vi "Handle Web service.vi"(7 "LabVIEW Web Service Request 2":refnum<class "Web Request.lvclass">, 11 "Server Name":string="3 phase testbench") -> ()   [LabVIEW 2025, in "MCP Server.lvlib"]
doc: "Use this VI in your LabVIEW Webservice inside a POST Method of any name. Just connect the Web Service reference, and the mcp server toolkit will handle all requests coming in through this method."
uses:
  MCP Server.lvlib
  <vilib>/wsapi/Web Request.lvclass
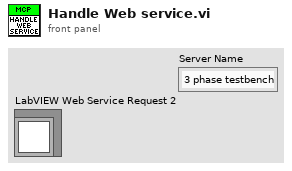
[diagram p1: front panel]
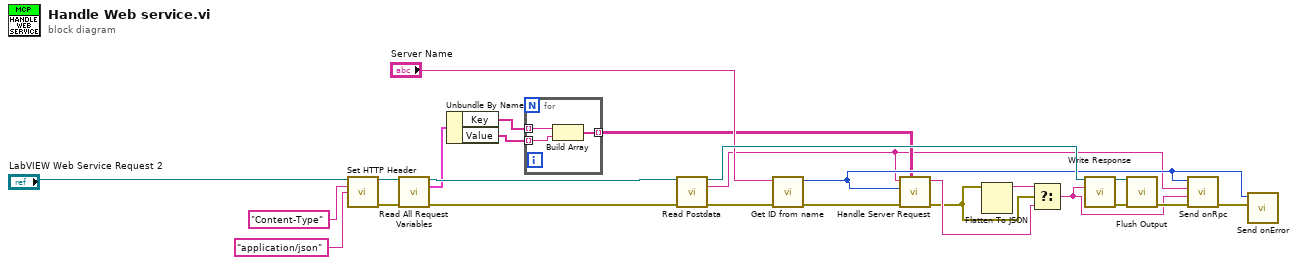
[diagram p0: block diagram]
diagram:
  n1 = call <vilib>:"Set HTTP Header.vi"("LabVIEW Web Service Request"="LabVIEW Web Service Request 2", "header"="Content-Type", "header value"="application/json") -> ("LabVIEW Web Service Request out"=w6:refnum<class "Web Request.lvclass">, "error out"=w9:errorcluster)  [unwired: 11 in]
  n2 = call <vilib>:"Read All Request Variables.vi"("LabVIEW Web Service Request"=w6, "error in (no error)"=w9) -> ("LabVIEW Web Service Request out"=w13:refnum<class "Web Request.lvclass">, "request variables"=w5:cluster{"Key":string[], "Value":string[]}, "error out"=w14:errorcluster)  [unwired: 11 in]
  n3 = Unbundle By Name(w5) -> ("Key"=w4:string[], "Value"=w3:string[])
  n4 = for {
    tunnel: [w28] -> w12 mode=indexing
    tunnel: w4 -> [w27] mode=indexing
    tunnel: w3 -> [w26] mode=indexing
    n5 = Build Array(w27, w26) -> (w28:string[])
  }
  n6 = call <vilib>:"Read Postdata.vi"("LabVIEW Web Service Request"=w13, "error in (no error)"=w14) -> ("LabVIEW Web Service Request out"=w25:refnum<class "Web Request.lvclass">, "postdata"=w2:string, "error out"=w16:errorcluster)  [unwired: 11 in]
  n7 = call "Get ID from name.vi"("error in (no error)"=w16, "Name"="Server Name") -> ("error out"=w17:errorcluster, "id out"=w23:i32)  [unwired: 7 in, 1 out]
  n8 = call "Handle Server Request.vi"("parameters"=w12, "error in (no error)"=w17, "id in"=w23, "request"=w2) -> ("error out"=w11:errorcluster, "response"=w18:string)  [unwired: 6 in]
  n9 = Flatten To JSON(anything=w11) -> (JSON string=w10:string)  [unwired: 2 in, 1 out]
  n10 = Select(t=w10, s=w11, f=w18) -> (s? t:f=w19:string)
  n11 = call <vilib>:"Write Response.vi"("LabVIEW Web Service Request"=w25, "response string"=w19) -> ("LabVIEW Web Service Request out"=w20:refnum<class "Web Request.lvclass">, "error out"=w21:errorcluster)  [unwired: 12 in]
  n12 = call <vilib>:"Flush Output.vi"("LabVIEW Web Service Request"=w20, "error in (no error)"=w21) -> ("error out"=w22:errorcluster)  [unwired: 12 in, 1 out]
  n13 = call "Send onRpc.vi"("error in (no error)"=w22, "response"=w19, "request"=w2, "id"=w23) -> ("error out"=w24:errorcluster)  [unwired: 7 in]
  n14 = call "Send onError.vi"("error to report"=w24, "id"=w23) -> ()  [unwired: 9 in, 1 out]
